vi "__toLowerCase.vi"(0 "Data Name in":string, 1 "to lowercase?(F)":bool) -> (5 "Data Name out":string)   [LabVIEW 2019, in "lv-apt-json-file.lvlib"]
uses:
  lv-apt-json-file.lvlib
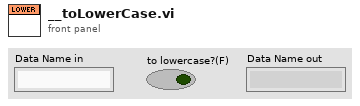
[diagram p1: front panel]
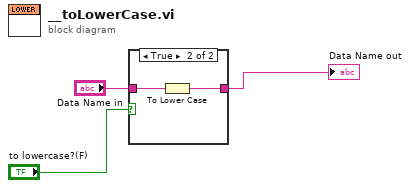
[diagram p0: block diagram]
diagram:
  n1 = case shown="True" "to lowercase?(F)" {
    tunnel: "Data Name in" -> [w4 w6]
    tunnel: [w4 w5] -> w2
    frame False {
    }
    frame True {
      n2 = To Lower Case(string=w6) -> (all lower case string=w5:string)
    }
  }
  "Data Name out" <- w2
